vi "2 - Use the NI-DAQmx VIs (Solution).vi"() -> ()   [LabVIEW 2013]
uses:
  <vilib>/DAQmx/read.llb/DAQmx Read (Analog 1D Wfm NChan NSamp).vi
  <vilib>/DAQmx/create/channels.llb/DAQmx Create Channel (AI-Temperature-Thermocouple).vi
  <vilib>/DAQmx/configure/timing.llb/DAQmx Timing (Sample Clock).vi
  <vilib>/DAQmx/miscellaneous.llb/DAQmx Fill In Error Info.vi
  <resource>/objmgr/daqmx.rc
panel:
  out "Alarm Output":bool
  in  "Alarm Level":dbl=26.0
  out "Temperature":waveform(dbl)[](graph)
  in  "stop":bool
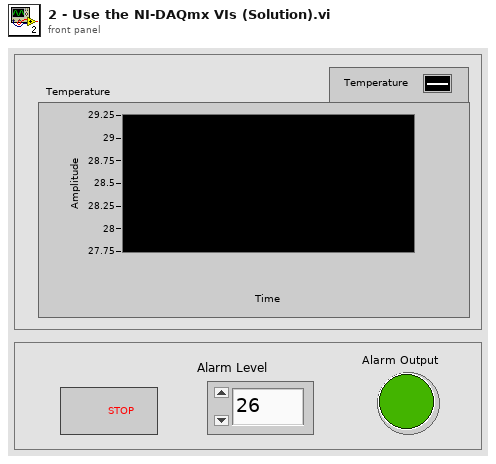
[diagram p1: front panel]
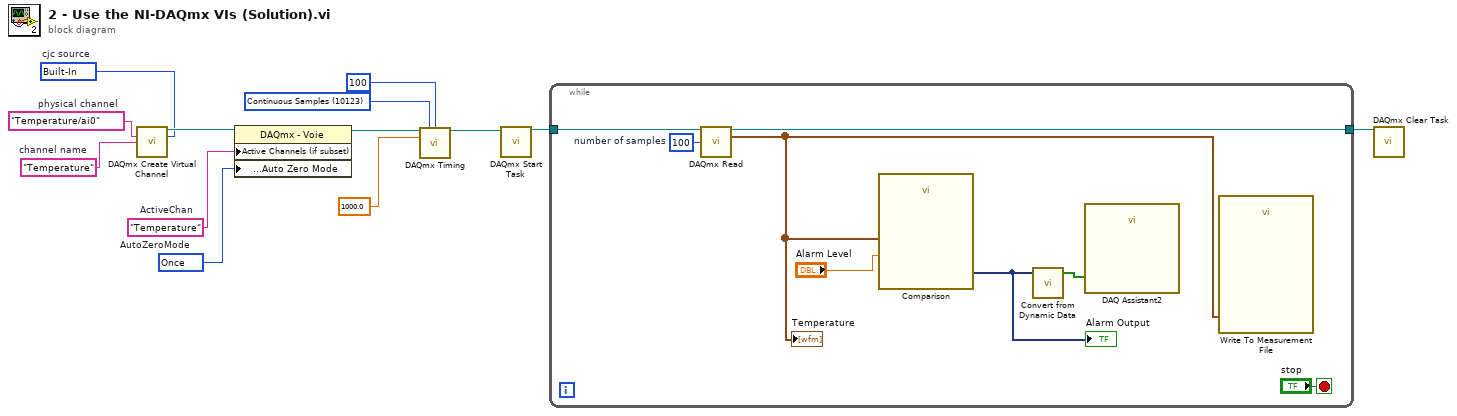
[diagram p0: block diagram]
diagram:
  w3 = 10123 items=["Finite Samples"=10178, "Continuous Samples"=10123, "Hardware Timed Single Point"=12522] ("sample mode")
  w6 = tag "Temperature/ai0"  # physical channel
  w8 = 10200 items=["Built-In"=10200, "Constant Value"=10116, "Channel"=10113]  # cjc source
  w7 = 10244 items=["None"=10230, "Once"=10244, "Every Sample"=10164]  # AutoZeroMode
  w9 = "Temperature"  # ActiveChan
  w11 = "Temperature"  # channel name
  n1 = call-poly <vilib>:"DAQmx Create Virtual Channel.vi"("physical channels"=w6, "cjc source"=w8, "name to assign"=w11) -> ("task out"=w10:refnum<k21>)  [unwired: 11 in, 1 out]
  n2 = property class="DAQmx - Voie"(reference=w10, "Active Channels (if subset)"=w9, "Analog Input:General Properties:Advanced:High Accuracy Settings:Auto Zero Mode"=w7) -> (reference out=w5:refnum<k21>)  [unwired: 1 in, 1 out]
  n3 = call-poly <vilib>:"DAQmx Timing.vi"("task/channels in"=w5, "sample mode"=w3, "samples per channel"=100, "rate"=1000.0) -> ("task out"=w4:refnum<k21>)  [unwired: 10 in, 1 out]
  n4 = call <vilib>:"DAQmx Start Task.vi"("task/channels in"=w4) -> ("task out"=w13:refnum<k21>)  [unwired: 13 in, 1 out]
  n5 = while {
    tunnel: w13 -> [w17]
    tunnel: [w16] -> w12
    stop <- "stop" stop-if-true
    w14 = 100  # number of samples
    n6 = call-poly <vilib>:"DAQmx Read.vi"("task/channels in"=w17, "number of samples per channel"=w14) -> ("task out"=w16:refnum<k21>, "data"=w15:waveform(dbl)[])  [unwired: 11 in, 1 out]
    "Temperature" <- w15
    n7 = call "Comparison"("Operand 2"="Alarm Level", "Operand 1"=w15) -> ("Result"=w19:dynamicdata)  [unwired: 1 in, 8 out]
    "Alarm Output" <- w19
    n8 = call "Convert from Dynamic Data"("Dynamic Data Type"=w19) -> ("Array"=w18:bool[])  [unwired: 3 in]
    n9 = call "DAQ Assistant2"("data"=w18) -> ()  [unwired: 4 in, 15 out]
    n10 = call "Write To Measurement File"("Signals"=w15) -> ()  [unwired: 16 in, 3 out]
  }
  n11 = call <vilib>:"DAQmx Clear Task.vi"("task in"=w12) -> ()  [unwired: 14 in, 1 out]
